vi "Output (String).vi"(8 "error in (no error)":errorcluster, 9 "position":cluster{"row":i8, "column":i8}, 10 "text":string, 11 "LCD in":refnum<class "Character LCD.lvclass">) -> (0 "error out":errorcluster, 1 "current cursor position":cluster{"row":i8, "column":i8}, 3 "LCD out":refnum<class "Character LCD.lvclass">)   [LabVIEW 2017, in "HD44780 Host.lvlib"]
doc: "Writes text strings or character codes on character LCD devices."
uses:
  HD44780 Host.lvlib
  Internal/LCD Class/Character LCD.lvclass
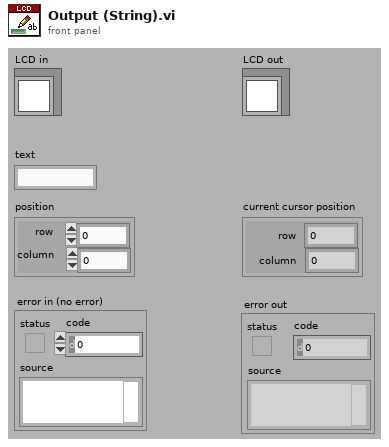
[diagram p1: front panel]
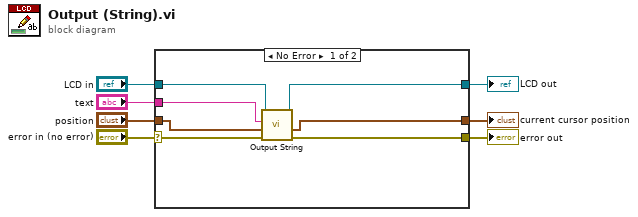
[diagram p0: block diagram]
diagram:
  n1 = case shown="No Error" "error in (no error)" {
    selector: "error in (no error)" -> [w13 w17]
    tunnel: [w14 w17] -> w6
    tunnel: "LCD in" -> [w10 w16]
    tunnel: [w9 w16] -> w4
    tunnel: "text" -> [w12 _]
    tunnel: "position" -> [w11 w15]
    tunnel: [w8 w15] -> w1
    frame No Error {
      n2 = call-dynamic "Output String.vi"("error in (no error)"=w13, "position"=w11, "text"=w12, "Character LCD in"=w10) -> ("error out"=w14:errorcluster, "current cursor position"=w8:cluster{"row":i8, "column":i8}, "Character LCD out"=w9:refnum<class "Character LCD.lvclass">)  [unwired: 5 in]
    }
    frame Error {
    }
  }
  "error out" <- w6
  "LCD out" <- w4
  "current cursor position" <- w1
